vi "DigitalOutput-Command string parser.vi"(0 "Command string":string) -> (2 "Pulse length (ms)":i32, 3 "Line index":i32, 4 "Drive high?":bool)   [LabVIEW 2015]
doc: "Parses a command string for the DigitalOutput output device.\n\"Continuous?\" indicates whether this is a switch (true) or pulse (false) operation\n\"Pulse length\" is the pulse length in ms, or 0 if it is a switch\n\"Line index\" is the index of which line to switch\n\"Drive high?\" indicates whether this is an on (true) of off (false) operation\n\nExample command strings:\npulse;0;on;30;\nswitch;3;off;"
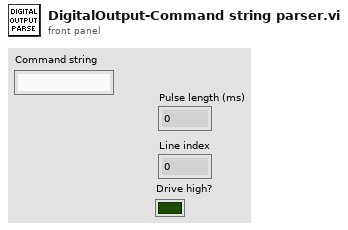
[diagram p1: front panel]
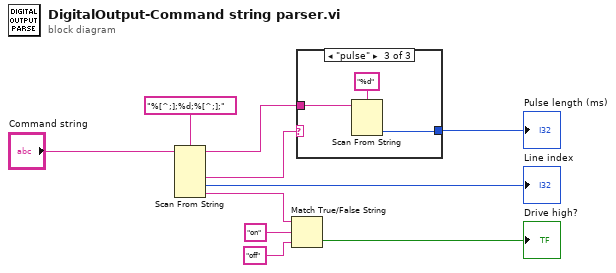
[diagram p0: block diagram]
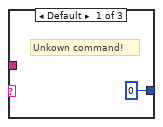
[diagram p2: hidden frame]
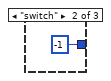
[diagram p3: hidden frame]
diagram:
  n1 = Scan From String(format string="%[^;];%d;%[^;];", input string="Command string") -> (remaining string=w9:string, output 1=w8:string, output 2=→"Line index":i32, output 3=w4:string)  [unwired: 5 in, 2 out]
  n2 = Match True/False String(2:"off" ("false string"), 3:"on" ("true string"), 4:w4) -> (0:→"Drive high?":bool)  [unwired: 1 out]
  n3 = case shown="\"pulse\"" w8 {
    tunnel: w9 -> [_ _ w14]
    tunnel: [0 -1 w13] -> w1
    frame Default {
      # "Unkown command!"
    }
    frame "switch" {
    }
    frame "pulse" {
      n4 = Scan From String(format string="%d", input string=w14) -> (output 1=w13:i32)  [unwired: 3 in, 3 out]
    }
  }
  "Pulse length (ms)" <- w1
